vi "createError.vi"(7 "ErrorCode":T1, 8 "error in":errorcluster, 11 "message":string) -> (0 "error out":errorcluster)   [LabVIEW 2013]
uses:
  Ctrls/EnumErrors.ctl
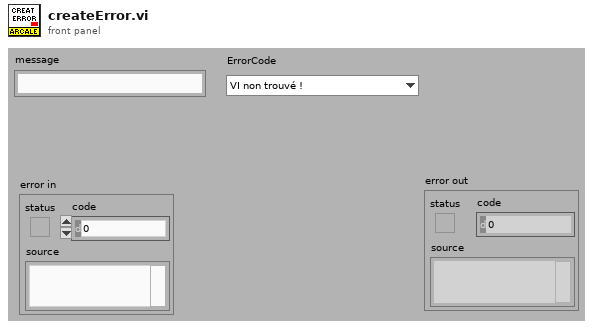
[diagram p1: front panel]
types:
  T1 = typedef "EnumErrors.ctl" = enum16{"VI non trouvé !", "Clé non trouvée", "Timeout", "Le VI tourne déjà", "Erreur de séparateur décimal", "Référence non trouvée"}
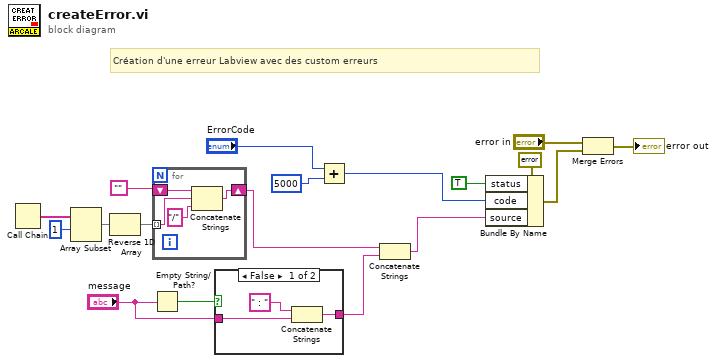
[diagram p0: block diagram]
diagram:
  # "Création d'une erreur Labview avec des custom erreurs"
  n1 = Call Chain() -> (call chain=w9:string[])
  n2 = Array Subset(array=w9, index=1) -> (w7:string[])  [unwired: 1 in]
  n3 = Reverse 1D Array(array=w7) -> (reversed array=w4:string[])
  n4 = Empty String/Path?(string/path="message") -> (empty?=w15:bool)
  n5 = for {
    tunnel: w4 -> [w20] mode=indexing
    shift-right: [w22] -> w5
    shift-left: "" -> [w21]
    n6 = Concatenate Strings(w21, w20, "/" ("string")) -> (w22:string)
  }
  n7 = case shown="False" w15 {
    tunnel: "message" -> [w24 w26]
    tunnel: [w25 w26] -> w13
    frame False {
      n8 = Concatenate Strings(" : " ("string"), w24) -> (w25:string)
    }
    frame True {
    }
  }
  n9 = Add(x="ErrorCode", y=5000) -> (x+y=w12:i32)
  n10 = Concatenate Strings(w5, w13) -> (w16:string)
  n11 = Bundle By Name(cluster=errorcluster {"status"=FALSE, "code"=0, "source"=""} ("error out"), "status"=TRUE, "code"=w12, "source"=w16) -> (w2:errorcluster)
  n12 = Merge Errors("error in", w2) -> (→"error out":errorcluster)
